vi "C4Buf_getNumParts.vi"(0 "c4buf in":refnum<k24>, 11 "error in (no error)":errorcluster) -> (4 "c4buf out":refnum<k24>, 6 "numParts out":i64, 15 "error out":errorcluster)   [LabVIEW 2015, in "libC4HdlLV.lvlib"]
uses:
  libC4HdlLV.lvlib
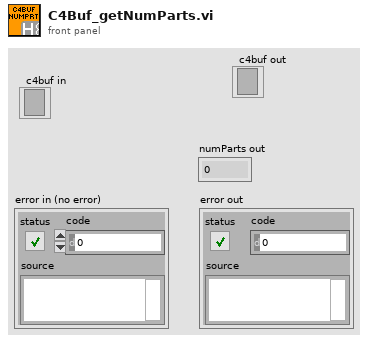
[diagram p1: front panel]
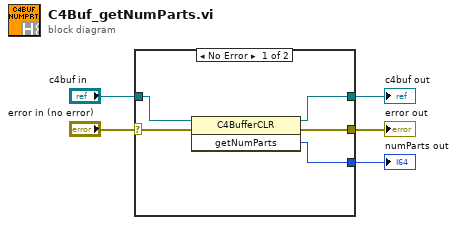
[diagram p0: block diagram]
diagram:
  n1 = case shown="No Error" "error in (no error)" {
    selector: "error in (no error)" -> [w9 w12]
    tunnel: [w8 w12] -> w4
    tunnel: "c4buf in" -> [w10 w11]
    tunnel: [w7 w11] -> w2
    tunnel: [w6 _] -> w1
    frame No Error {
      n2 = invoke class="C4BufferCLR" method="getNumParts"(reference=w10, error in=w9) -> (reference out=w7:refnum<k24>, error out=w8:errorcluster, "getNumParts"=w6:i64)  [unwired: 1 in]
    }
    frame Error {
    }
  }
  "error out" <- w4
  "c4buf out" <- w2
  "numParts out" <- w1
